vi "MeasureIVandCap.vi"(0 ".NET Refnum in":refnum<k24>, 1 ".NET Refnum":refnum<k24>, 2 "Junction Name":string, 7 "appended path":path, 9 "Numeric":dbl, 12 "new file path (Not A Path if cancelled)":path, 13 "UiDefinition":T1, 14 "Function":string) -> (15 "error out":errorcluster)   [LabVIEW 2020]
uses:
  D:/LabviewDXFViewer/LabviewDXFViewer/bin/Release/LabviewDXFViewer.exe
  LabviewDXFViewer/bin/Release/LabviewDXFViewer.exe
  UIReferences.ctl
  <vilib>/Utility/file.llb/Write Delimited Spreadsheet (DBL).vi
  <vilib>/Utility/file.llb/Write Delimited Spreadsheet (string).vi
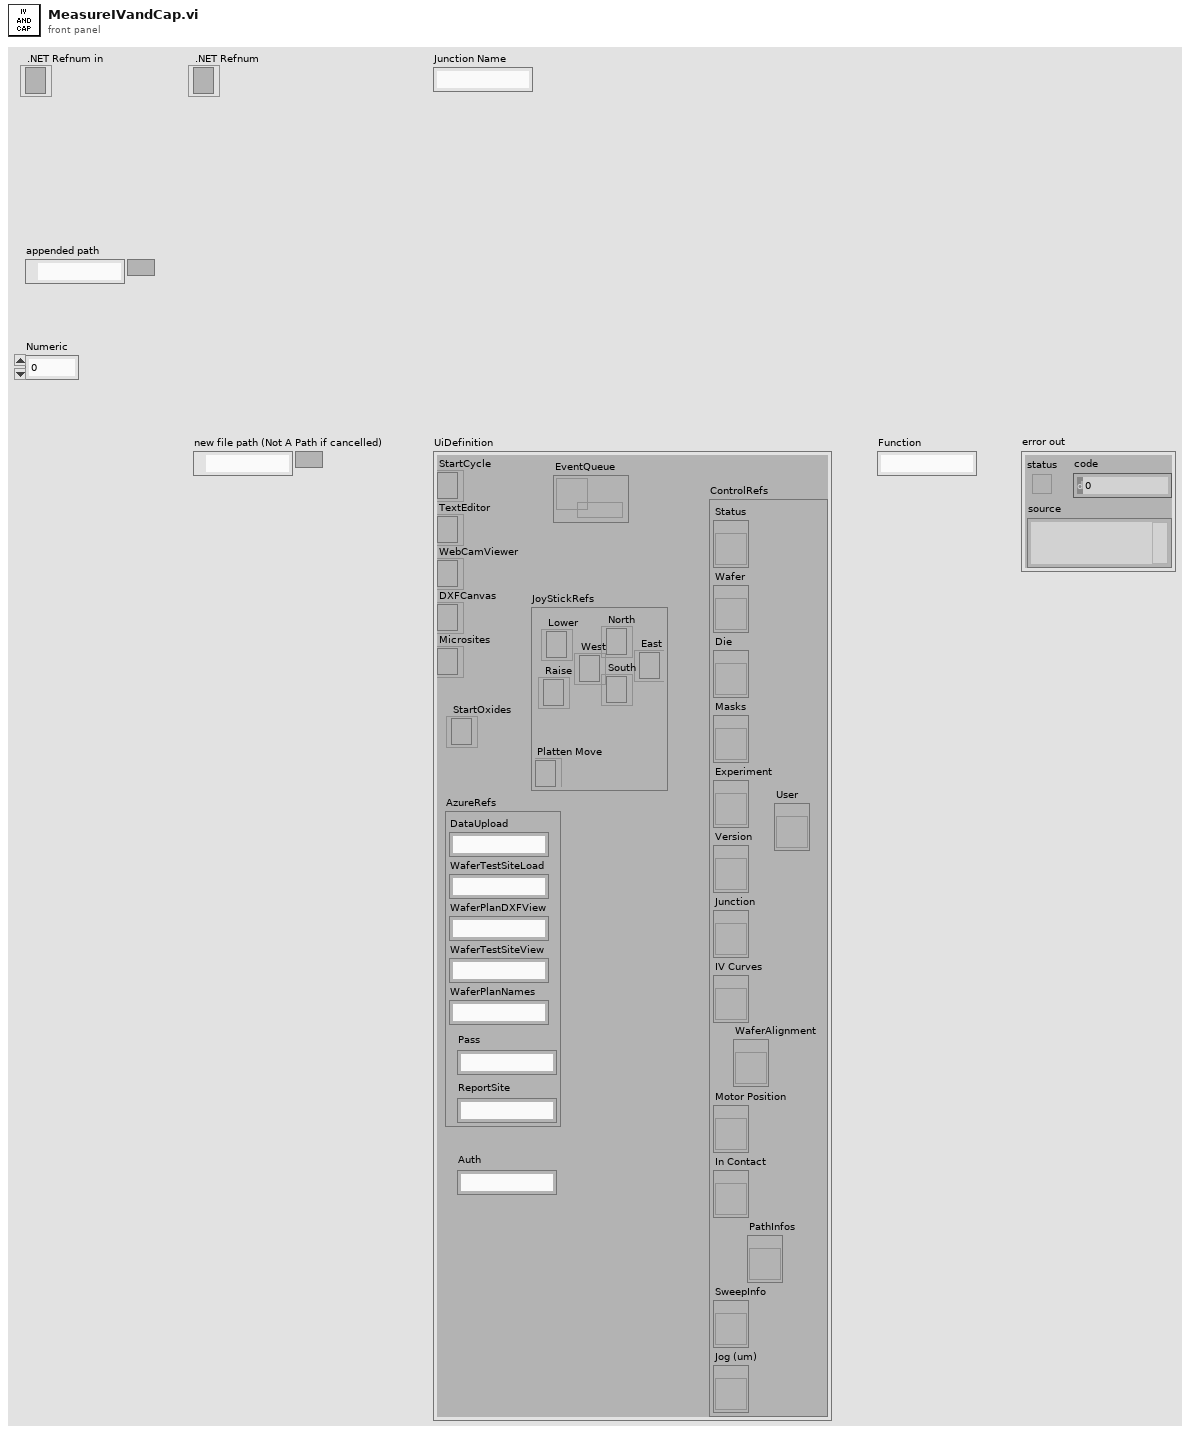
[diagram p1: front panel]
types:
  T1 = typedef "UIReferences.ctl" = cluster{"StartCycle":refnum<k24>, "TextEditor":refnum<k24>, "WebCamViewer":refnum<k24>, "DXFCanvas":refnum<k24>, "Microsites":refnum<k24>, "JoyStickRefs":cluster{"North":refnum<k24>, "Lower":refnum<k24>, "Raise":refnum<k24>, "Platten Move":refnum<k24>, "West":refnum<k24>, "East":refnum<k24>, "South":refnum<k24>}, "AzureRefs":cluster{"DataUpload":string, "WaferTestSiteLoad":string, "WaferPlanDXFView":string, "WaferTestSiteView":string, "WaferPlanNames":string, "Pass":string, "ReportSite":string}, "ControlRefs":cluster{"Status":refnum<vi>, "Wafer":refnum<vi>, "Die":refnum<vi>, "Masks":refnum<vi>, "Experiment":refnum<vi>, "Version":refnum<vi>, "Junction":refnum<vi>, "IV Curves":refnum<vi>, "Motor Position":refnum<vi>, "In Contact":refnum<vi>, "SweepInfo":refnum<vi>, "Jog (um)":refnum<vi>, "PathInfos":refnum<vi>, "User":refnum<vi>, "WaferAlignment":refnum<vi>}, "EventQueue":refnum<queue>, "StartOxides":refnum<k24>, "Auth":string}
  T2 = typedef "CapacitanceInfos.ctl" = cluster{"Conductance":dbl, "CapacitanceIV":dbl, "Intercept":dbl, "CapacitanceSW":dbl, "Sum":dbl, "CapacitanceInfos":T3[], "CapacitancePhase":dbl, "dC/dV":dbl, "Function":string, "OtherInfo":dbl[][]}
  T3 = typedef "CapacitanceRecord.ctl" = cluster{"Freq":dbl, "Vpp":dbl, "PhaseS":dbl, "Irms":dbl, "PhaseC":dbl, "Theta":dbl, "VDrive":dbl, "Capacitance":dbl, "Other":dbl}
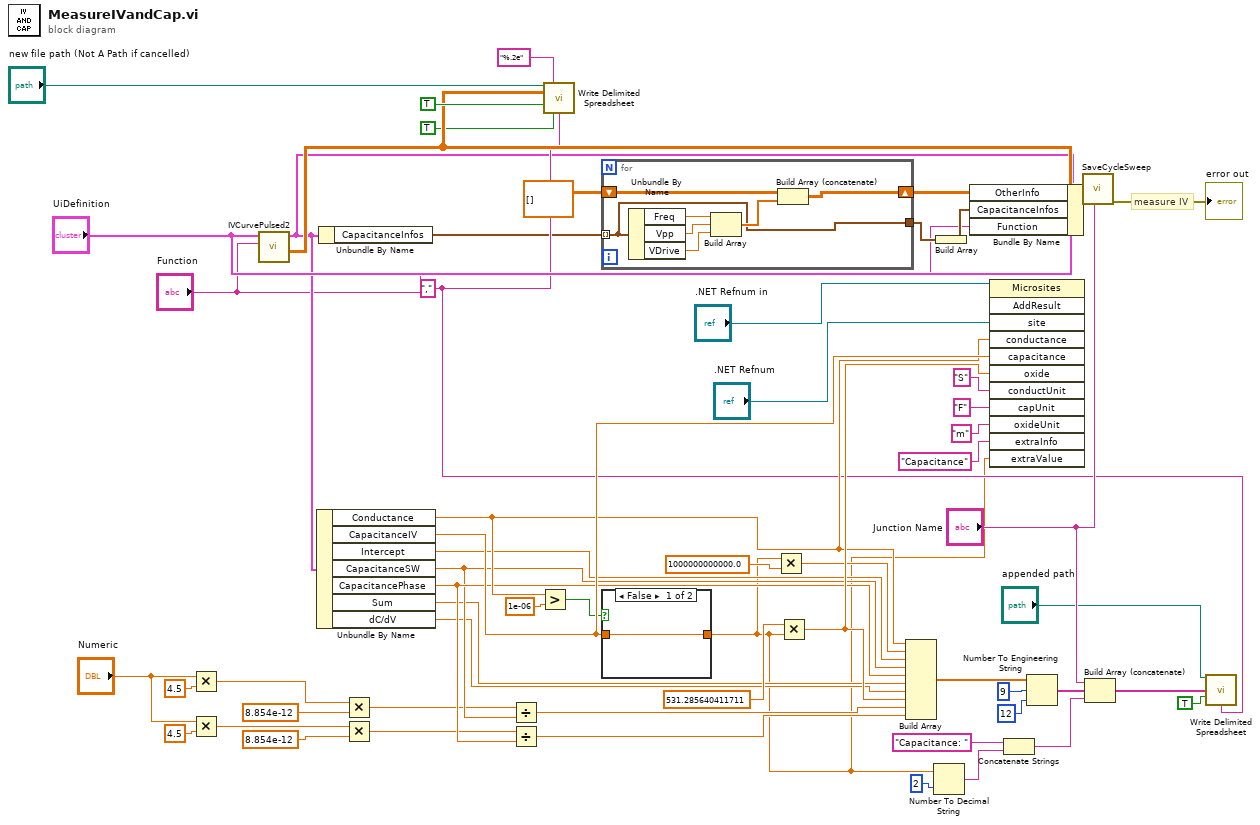
[diagram p0: block diagram]
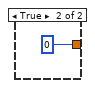
[diagram p2: hidden frame]
diagram:
  w15 = "," ("delimiter (\\t)")
  # "measure IV"
  n1 = Multiply(x="Numeric", y=4.5) -> (x*y=w36:dbl)
  n2 = Multiply(x="Numeric", y=4.5) -> (x*y=w42:dbl)
  n3 = call "IVCurvePulsed2.vi"("Program"="Function", "UiDefinition"="UiDefinition") -> ("appended array"=w26:dbl[][], "InfoCluster"=w8:T2)  [unwired: 8 in]
  n4 = Unbundle By Name(w8) -> ("Conductance"=w56:dbl, "CapacitanceIV"=w57:dbl, "Intercept"=w30:dbl, "CapacitanceSW"=w39:dbl, "CapacitancePhase"=w46:dbl, "Sum"=w31:dbl, "dC/dV"=w32:dbl)
  n5 = Unbundle By Name(w8) -> ("CapacitanceInfos"=w7:T3[])
  n6 = Multiply(x=w36, y=8.854e-12) -> (x*y=w38:dbl)
  n7 = Multiply(x=w42, y=8.854e-12) -> (x*y=w44:dbl)
  n8 = Divide(x=w38, y=w39) -> (x/y=w40:dbl)
  n9 = Divide(x=w44, y=w46) -> (x/y=w47:dbl)
  n10 = Greater?(x=w56, y=1e-06) -> (0:w48:bool)
  n11 = call-poly <vilib>:"Write Delimited Spreadsheet.vi"("file path (dialog if empty)"="new file path (Not A Path if cancelled)", "format (%.3f)"="%.2e", "2D data"=w26, "append to file? (new file:F)"=TRUE, "transpose? (no:F)"=TRUE, "delimiter (\\t)"=w15) -> ()  [unwired: 8 in, 2 out]
  n12 = for {
    tunnel: w7 -> [w60] mode=indexing
    shift-right: [w62] -> w4
    shift-left: dbl[][] [] -> [w61]
    tunnel: [w60] -> w3
    n13 = Unbundle By Name(w60) -> ("Freq"=w66:dbl, "Vpp"=w65:dbl, "VDrive"=w64:dbl)
    n14 = Build Array(w66, w65, w64) -> (w63:dbl[])
    n15 = Build Array (concatenate)(w61, w63) -> (w62:dbl[][])
  }
  n16 = case shown="False" w48 {
    tunnel: [w67 0] -> w11
    tunnel: w57 -> [w67 _]
    frame False {
    }
    frame True {
    }
  }
  n17 = Multiply(x=w11, y=1000000000000.0) -> (x*y=w33:dbl)
  n18 = Multiply(x=531.285640411711, y=w11) -> (x*y=w59:dbl)
  n19 = Build Array(w56, w33, w30, w39, w46, w31, w32, w59, w40, w47) -> (w29:dbl[])
  n20 = Number To Decimal String(number=w11, width (-)=i16 2) -> (decimal integer string=w13:string)
  n21 = Build Array(w3) -> (w2:T3[])
  n22 = Bundle By Name(cluster=w8, "OtherInfo"=w4, "CapacitanceInfos"=w2, "Function"="Function") -> (w5:T2)
  n23 = invoke class="Microsites" method="AddResult"(reference=".NET Refnum in", "site"=".NET Refnum", "conductance"=w56, "capacitance"=w57, "oxide"=w59, "conductUnit"="S", "capUnit"="F", "oxideUnit"="m" ("interceptUnit"), "extraInfo"="Capacitance", "extraValue"=w11) -> ()  [unwired: 2 in, 12 out]
  n24 = Concatenate Strings("Capacitance: ", w13) -> (w9:string)
  n25 = Number To Engineering String(2:i16 12 ("precision (6)"), 3:i16 9 ("width (-)"), 4:w29) -> (0:w20:string[])  [unwired: 1 in]
  n26 = call "SaveCycleSweep.vi"("JunctionName"="Junction Name", "UiDefinition 2"="UiDefinition", "InfoCluster"=w5, "appended array"=w26) -> ("error out"=→"error out":errorcluster)  [unwired: 7 in]
  n27 = Build Array (concatenate)("Junction Name", w20, w9) -> (w22:string[])
  n28 = call-poly <vilib>:"Write Delimited Spreadsheet.vi"("file path (dialog if empty)"="appended path", "1D data"=w22, "append to file? (new file:F)"=TRUE, "delimiter (\\t)"=w15) -> ()  [unwired: 10 in, 2 out]
